vi "all_stages - state_machine.vi"() -> ()   [LabVIEW 2024]
uses:
  O:/DSG/Tyler/EIC/DIRC/daq/automated/Thorlabs.MotionControl.Controls.dll
  Thorlabs.MotionControl.Controls.dll
  O:/DSG/Tyler/EIC/DIRC/daq/automated/Thorlabs.MotionControl.IntegratedStepperMotorsCLI.dll
  Thorlabs.MotionControl.IntegratedStepperMotorsCLI.dll
  O:/DSG/Tyler/EIC/DIRC/daq/automated/Thorlabs.MotionControl.Benchtop.StepperMotorCLI.dll
  Thorlabs.MotionControl.Benchtop.StepperMotorCLI.dll
  <instrlib>/Keithley 6517/Keithley 6517.lvlib
panel:
  out "main-stage-refs":T1
  out "state-queue":T2(array[cluster])
  in  "build-seq":bool
  in  "PDA":dbl=85.0 format="%#_13g"
  in  "BMA":dbl=45.0 format="%#_13g"
  in  "BarY":dbl=150.0 format="%#_13g"
  in  "BarX":dbl=300.0 format="%#_13g"
  in  "PDY":dbl=150.0 format="%#_13g"
  in  "PDX":dbl=300.0 format="%#_13g"
  out "bypass-confirm":bool
  out "ySeq_hist":dbl[][](array[numeric])
  out "xSeq_hist":dbl[][](array[numeric])
  out "xSeq_diff":dbl[](array[numeric])
  out "ySeq_diff":dbl[](array[numeric])
  out "ySeq_in":dbl[](array[numeric])
  out "xSeq_in":dbl[](array[numeric])
  out "ySeq_res":dbl[](array[numeric])
  out "xSeq_res":dbl[](array[numeric])
  in  "go_seq_test":bool
  out "PD Values":cluster{"PD1":dbl, "PD2":dbl, "PD3":dbl}
  out "last-PD":dbl[](array[numeric])=[1.0, 1.0, 1.0]
  in  "move-bar":bool
  in  "mode-select":T3(radio) caption="Mode Select"
  in  "auto-align-grid":bool
  in  "auto-delta":dbl=0.5
  out "max value":dbl
  out "xOut":dbl
  out "yOut":dbl
  out "max indexes":i32[](array[numeric])
  in  "k":dbl=25.0
  in  "N trials":dbl=16.0
  in  "auto-align":bool
  out "pd_angle":dbl
  out "brewster_angle":dbl
  out "meter-visa":refnum<visa-resource-name>
  out "loop-rate":u32
  out "meter-stat":bool caption="Log Status"
  out "file-stat":bool caption="Log Status"
  out "stage-stat":bool caption="Log Status"
  out "last-save-time":string caption="Time of Last Save:"
  out "pd_y_pos":dbl
  out "pd_x_pos":dbl
  out "bar_y_pos":dbl
  out "bar_x_pos":dbl
  in  "nSamples":dbl=50.0 caption="# Samples"
  out "Current Time:":string
  in  "save-data":bool
  in  "bar-note":bool
  out "pd3_v":dbl caption="PD 3" format="%#.4g"
  out "pd2_v":dbl caption="PD 2" format="%#.4g"
  out "pd1_v":dbl caption="PD 1" format="%#.4g"
  out "meter-error":errorcluster
  out "log-error":errorcluster
  out "log-path":path caption="Path Data Will Save To:"
  out "start-msg":string
  out "stage-error":errorcluster
  in  "PD Angle":refnum<k24>(container)
  in  "Brewster":refnum<k24>(container)
  in  "PD Y":refnum<k24>(container)
  in  "PD X":refnum<k24>(container)
  in  "BAR Y":refnum<k24>(container)
  in  "stop":bool
  in  "BAR X":refnum<k24>(container)
  out "pd-plt":cluster{"[0]":dbl, "[1]":dbl, "[2]":dbl}(graph) caption="Measurement History"
  # "EXPERT DEBUGGING INFO"
  # "A"
  # "A"
  # "A"
  # "Work In Progress - please do not use"
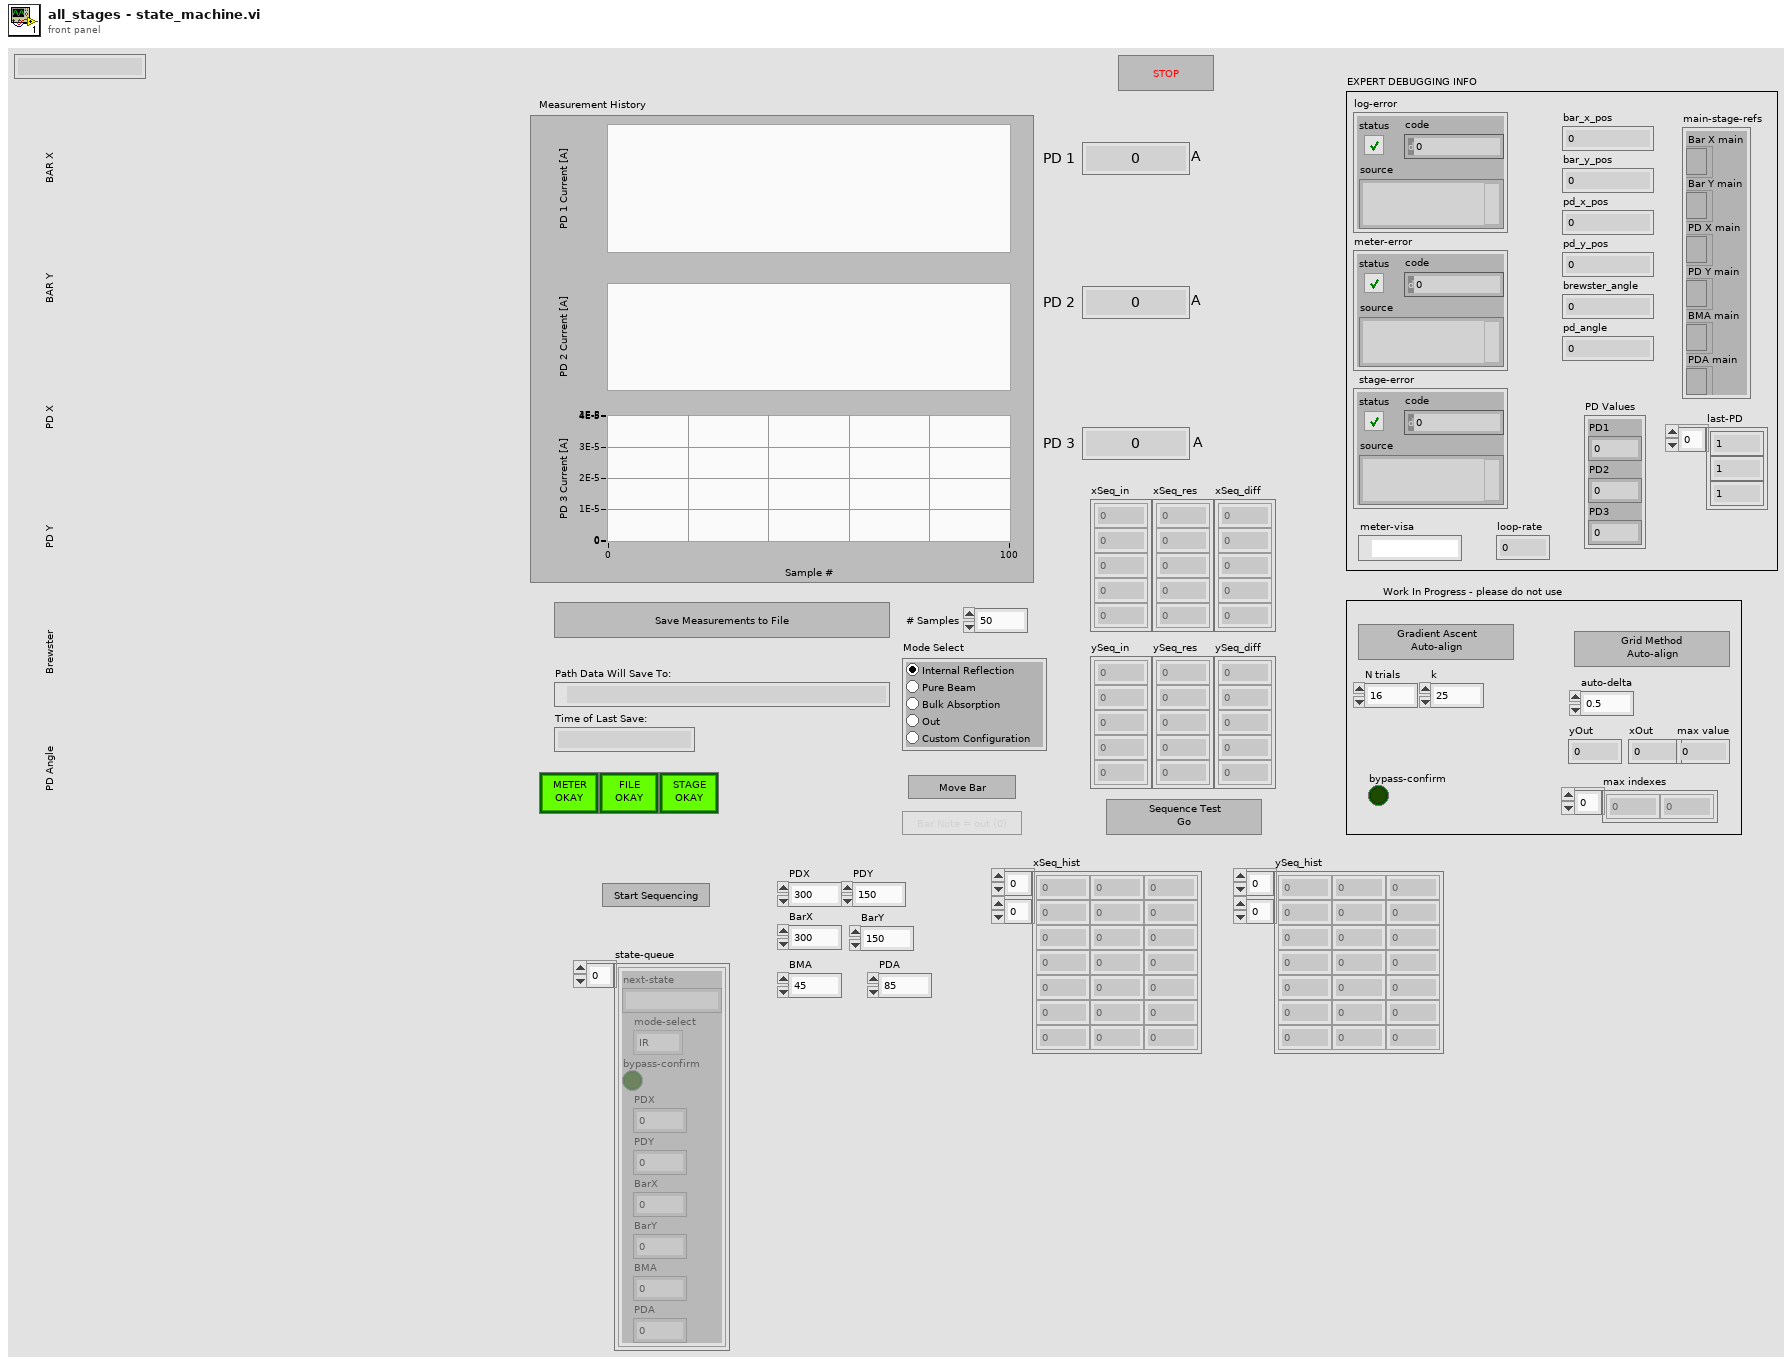
[diagram p1: front panel]
types:
  T1 = cluster{"Bar X main":refnum<k24>, "Bar Y main":refnum<k24>, "PD X main":refnum<k24>, "PD Y main":refnum<k24>, "BMA main":refnum<k24>, "PDA main":refnum<k24>}
  T2 = cluster{"next-state":string, "mode-select":enum32{"IR", "Pure", "Bulk", "Bar Out", "custom"}, "bypass-confirm":bool, "PDX":dbl, "PDY":dbl, "BarX":dbl, "BarY":dbl, "BMA":dbl, "PDA":dbl}[]
  T3 = enum32{"IR", "Pure", "Bulk", "Bar Out", "custom"}
  T4 = cluster{"Bar X":refnum<k24>, "Bar Y":refnum<k24>, "PD X":refnum<k24>, "PD Y":refnum<k24>, "Brewster":refnum<k24>, "PD Angle":refnum<k24>}
  T5 = enum16{"open", "replace", "create", "open or create", "replace or create", "replace or create with confirmation"}
  T6 = cluster{"next-state":string, "mode-select":enum32{"IR", "Pure", "Bulk", "Bar Out", "custom"}, "bypass-confirm":bool, "PDX":dbl, "PDY":dbl, "BarX":dbl, "BarY":dbl, "BMA":dbl, "PDA":dbl}
  T7 = cluster{"error":bool, "code":i32, "source":string}
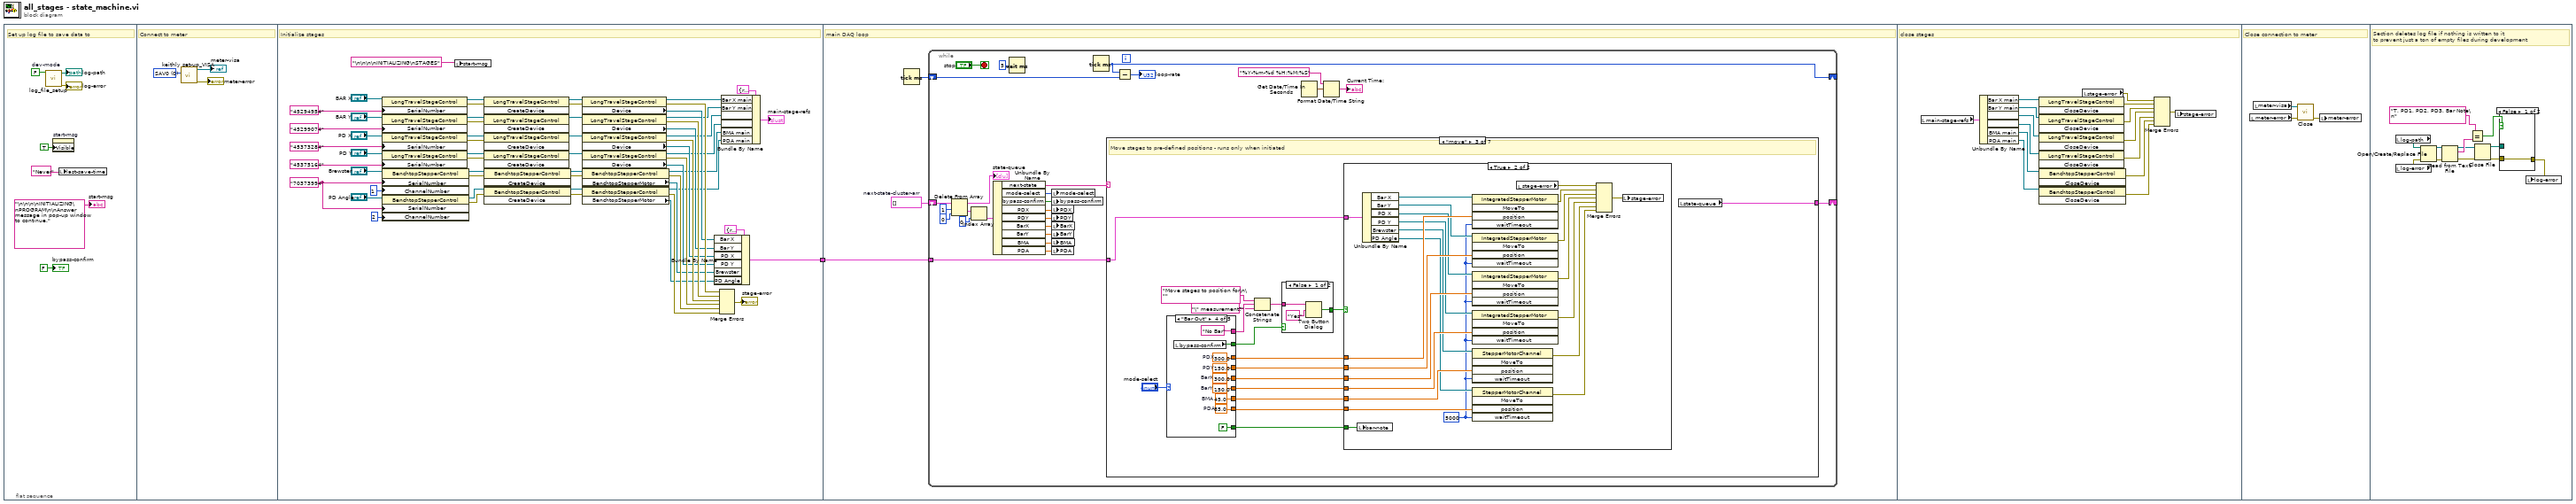
[diagram p0: block diagram]
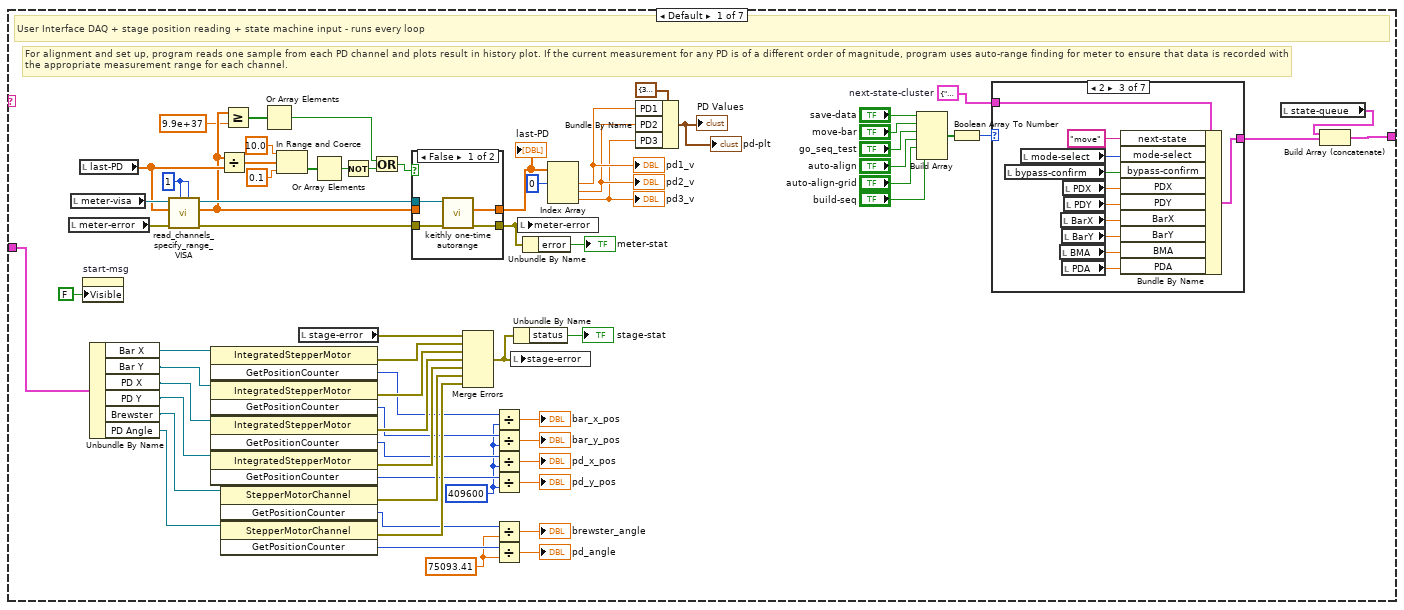
[diagram p2: hidden frame]
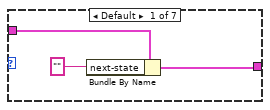
[diagram p3: hidden frame]
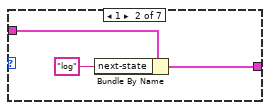
[diagram p4: hidden frame]
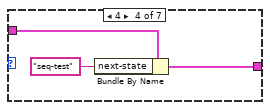
[diagram p5: hidden frame]
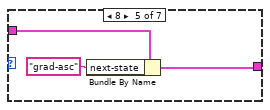
[diagram p6: hidden frame]
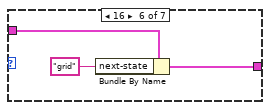
[diagram p7: hidden frame]
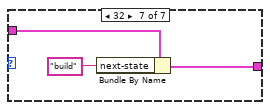
[diagram p8: hidden frame]
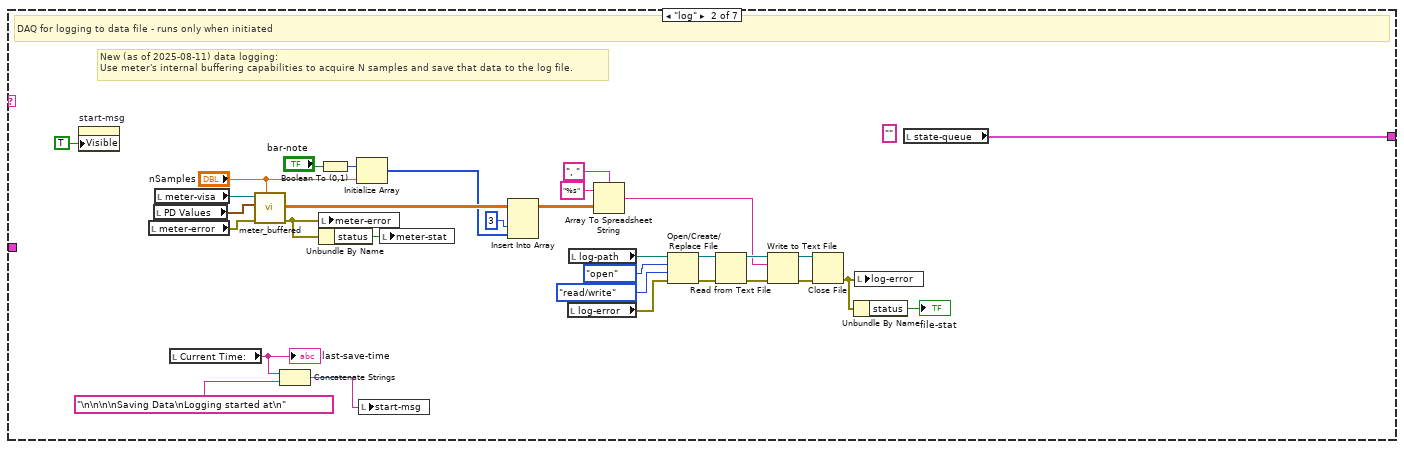
[diagram p10: hidden frame]
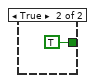
[diagram p11: hidden frame]
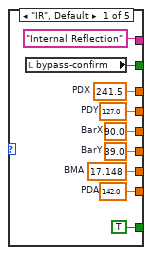
[diagram p12: hidden frame]
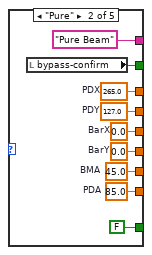
[diagram p13: hidden frame]
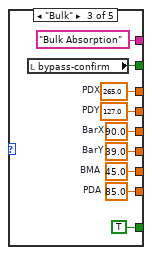
[diagram p14: hidden frame]
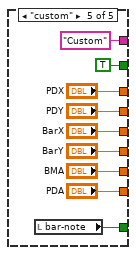
[diagram p15: hidden frame]
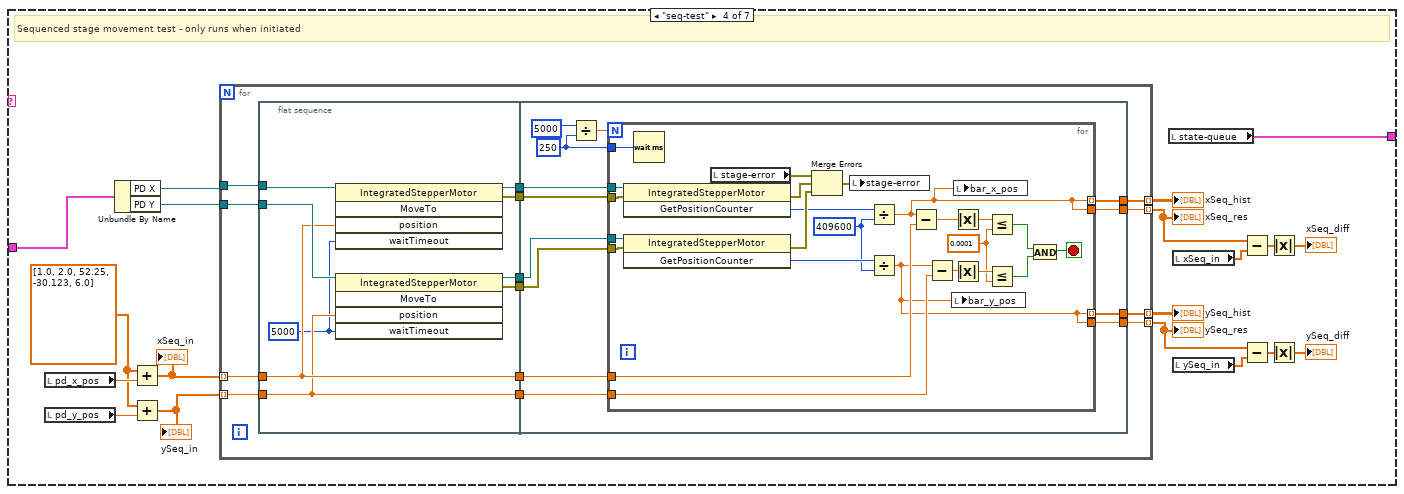
[diagram p17: hidden frame]
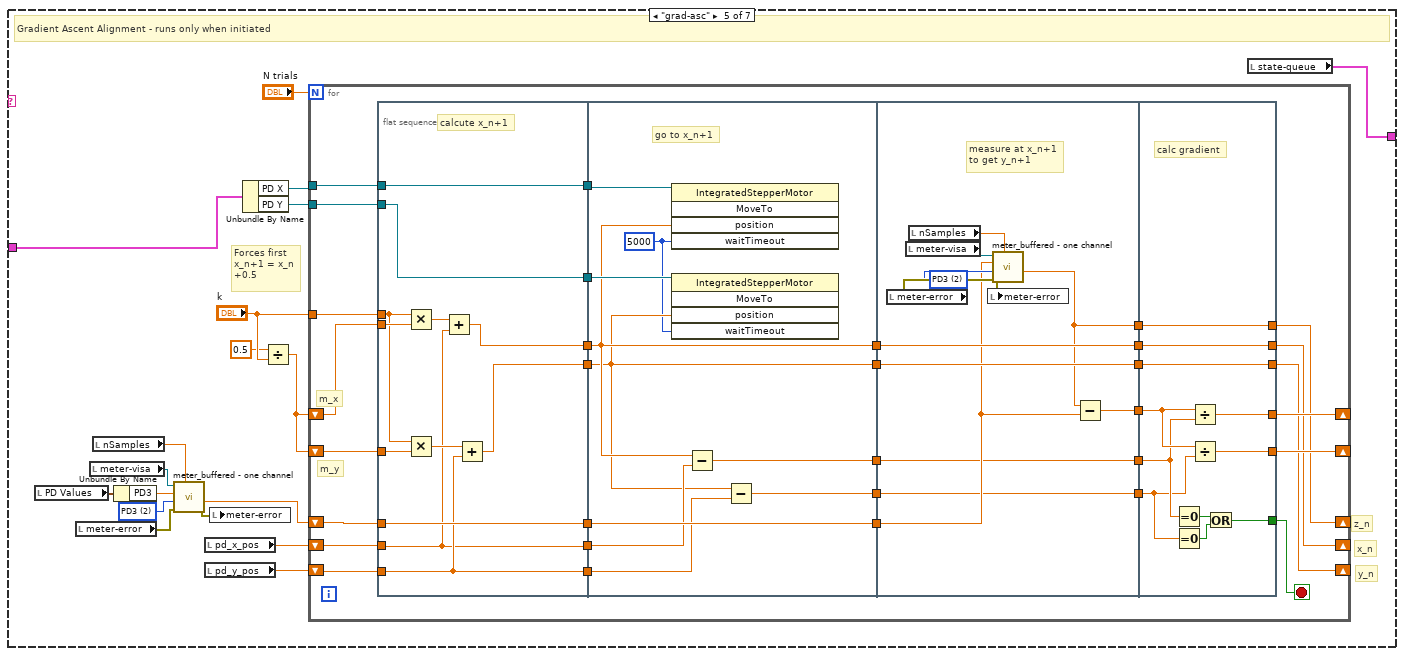
[diagram p18: hidden frame]
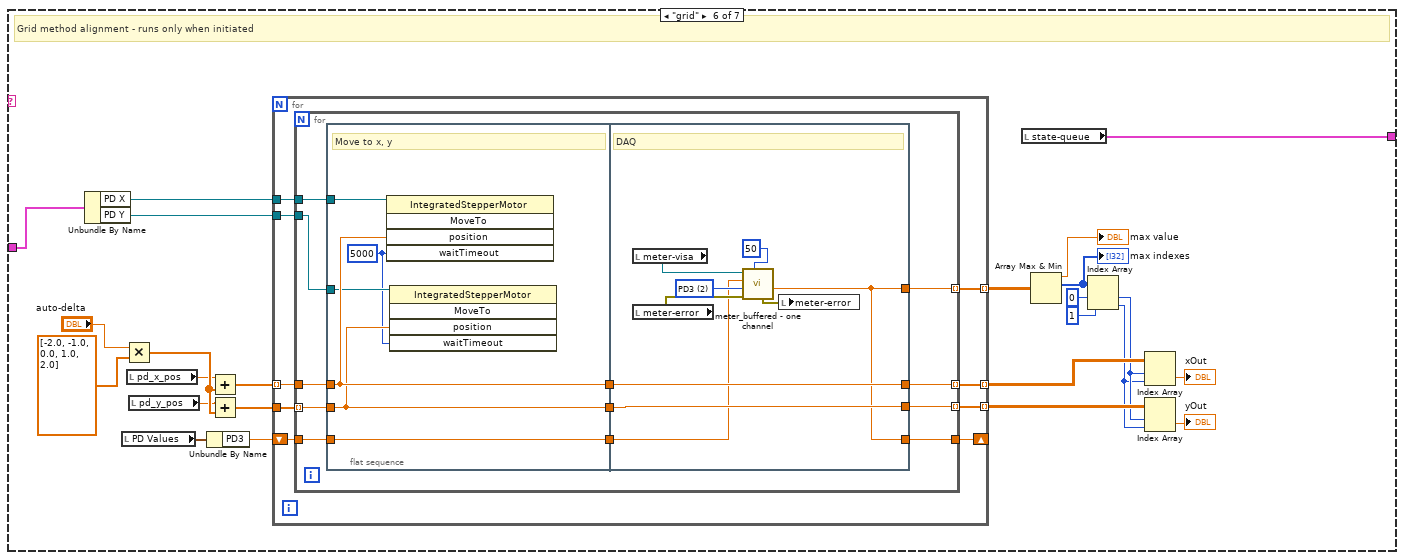
[diagram p19: hidden frame]
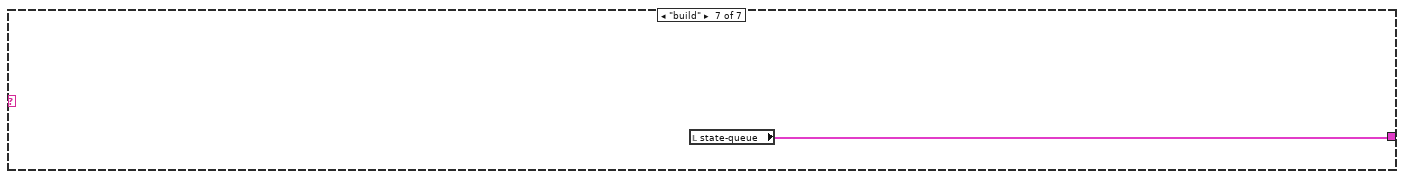
[diagram p20: hidden frame]
diagram:
  n1 = flat-sequence {
    tunnel: [w20] -> w1
    tunnel: w1 -> [w71]
    frame #0 {
      w8 = FALSE  # dev-mode
      # "Set up log file to save data to"
      n2 = call "log_file_setup.vi"("dev-mode"=w8) -> ("error out"=→"log-error":errorcluster, "appended path"=→"log-path":path)  [unwired: 8 in, 1 out]
      n3 = property on="start-msg" class="Str"("Visible"=TRUE) -> ()  [unwired: 2 in, 2 out]
      n4 = local write "last-save-time"("Never" ("date/time string")) -> ()
      "start-msg" <- "\n\n\n\nINITIALIZING\nPROGRAM\n\nAnswer message in pop-up window to continue." ("String")
      "bypass-confirm" <- FALSE
    }
    frame #1 {
      w9 = i16 0 items=["SAV0", "SAV1", "SAV2", "SAV3", "SAV4", "SAV5", "SAV6", "SAV7", "SAV8", "SAV9", "RST", "Preset"] ("ConfigOpt")
      # "Connect to meter"
      n5 = call "keithly set-up_VISA.vi"("ConfigOpt"=w9) -> ("error out"=→"meter-error":errorcluster, "meter-VISA"=→"meter-visa":refnum<visa-resource-name>)  [unwired: 9 in]
    }
    frame #2 {
      w28 = "70373994" ("SerialNumber")
      # "Initialize stages"
      n6 = property class="LongTravelStageControl"(reference="BAR X", "SerialNumber"="45294954") -> (reference out=w31:refnum<k24>, error out=w38:errorcluster)  [unwired: 1 in]
      n7 = property class="LongTravelStageControl"(reference="BAR Y", "SerialNumber"="45299074") -> (reference out=w32:refnum<k24>, error out=w39:errorcluster)  [unwired: 1 in]
      n8 = property class="LongTravelStageControl"(reference="PD X", "SerialNumber"="45373284") -> (reference out=w35:refnum<k24>, error out=w40:errorcluster)  [unwired: 1 in]
      n9 = property class="LongTravelStageControl"(reference="PD Y", "SerialNumber"="45375164") -> (reference out=w36:refnum<k24>, error out=w41:errorcluster)  [unwired: 1 in]
      n10 = property class="BenchtopStepperControl"(reference="Brewster", "SerialNumber"=w28, "ChannelNumber"=1) -> (reference out=w54:refnum<k24>, error out=w55:errorcluster)  [unwired: 1 in]
      n11 = property class="BenchtopStepperControl"(reference="PD Angle", "SerialNumber"=w28, "ChannelNumber"=2) -> (reference out=w53:refnum<k24>, error out=w56:errorcluster)  [unwired: 1 in]
      n12 = local write "start-msg"("\n\n\n\nINITIALIZING\nSTAGES" ("String")) -> ()
      n13 = invoke class="LongTravelStageControl" method="CreateDevice"(reference=w31, error in=w38) -> (reference out=w44:refnum<k24>, error out=w48:errorcluster)  [unwired: 1 in, 1 out]
      n14 = invoke class="LongTravelStageControl" method="CreateDevice"(reference=w32, error in=w39) -> (reference out=w45:refnum<k24>)  [unwired: 1 in, 2 out]
      n15 = invoke class="LongTravelStageControl" method="CreateDevice"(reference=w35, error in=w40) -> (reference out=w46:refnum<k24>)  [unwired: 1 in, 2 out]
      n16 = invoke class="LongTravelStageControl" method="CreateDevice"(reference=w36, error in=w41) -> (reference out=w47:refnum<k24>)  [unwired: 1 in, 2 out]
      n17 = invoke class="BenchtopStepperControl" method="CreateDevice"(reference=w54, error in=w55) -> (reference out=w51:refnum<k24>, error out=w49:errorcluster)  [unwired: 1 in, 1 out]
      n18 = invoke class="BenchtopStepperControl" method="CreateDevice"(reference=w53, error in=w56) -> (reference out=w50:refnum<k24>, error out=w52:errorcluster)  [unwired: 1 in, 1 out]
      n19 = property class="LongTravelStageControl"(reference=w44, error in=w48) -> (reference out=w18:refnum<k24>, error out=w68:errorcluster, "Device"=w57:refnum<k24>)
      n20 = property class="LongTravelStageControl"(reference=w45) -> (reference out=w17:refnum<k24>, error out=w63:errorcluster, "Device"=w58:refnum<k24>)  [unwired: 1 in]
      n21 = property class="LongTravelStageControl"(reference=w46) -> (reference out=w16:refnum<k24>, error out=w64:errorcluster, "Device"=w59:refnum<k24>)  [unwired: 1 in]
      n22 = property class="LongTravelStageControl"(reference=w47) -> (reference out=w15:refnum<k24>, error out=w65:errorcluster, "Device"=w60:refnum<k24>)  [unwired: 1 in]
      n23 = property class="BenchtopStepperControl"(reference=w51, error in=w49) -> (reference out=w14:refnum<k24>, error out=w66:errorcluster, "BenchtopStepperMotor"=w61:refnum<k24>)
      n24 = property class="BenchtopStepperControl"(reference=w50, error in=w52) -> (reference out=w13:refnum<k24>, error out=w67:errorcluster, "BenchtopStepperMotor"=w62:refnum<k24>)
      n25 = Bundle By Name(cluster=T4 {"Bar X"=refnum, "Bar Y"=refnum, "PD X"=refnum, "PD Y"=refnum, "Brewster"=refnum, "PD Angle"=refnum}, "Bar X"=w57, "Bar Y"=w58, "PD X"=w59, "PD Y"=w60, "Brewster"=w61, "PD Angle"=w62) -> (w20:T4)
      n26 = Merge Errors(w68, w63, w64, w65, w66, w67) -> (→"stage-error":errorcluster)
      n27 = Bundle By Name(cluster=T1 {"Bar X main"=refnum, "Bar Y main"=refnum, "PD X main"=refnum, "PD Y main"=refnum, "BMA main"=refnum, "PDA main"=refnum}, "Bar X main"=w18, "Bar Y main"=w17, "PD X main"=w16, "PD Y main"=w15, "BMA main"=w14, "PDA main"=w13) -> (→"main-stage-refs":T1)
    }
    frame #3 {
      w70 = T2 []  # next-state-cluster-arr
      # "main DAQ loop"
      n28 = Tick Count (ms)() -> (millisecond timer value=w72:u32)
      n29 = while {
        shift-right: [w97] -> _
        shift-left: w72 -> [w96]
        tunnel: w71 -> [w94]
        shift-right: [w73] -> _
        shift-left: w70 -> [w76]
        stop <- "stop" stop-if-true
        n30 = Delete From Array(array=w76, length=1, index=0) -> (deleted portion=w74:T2, array with subset deleted=→"state-queue":T2)
        n31 = Index Array(array=w74, index=0) -> (element=w86:T6)
        n32 = Unbundle By Name(w86) -> ("next-state"=w85:string, "mode-select"=w77:T3, "bypass-confirm"=w78:bool, "PDX"=w84:dbl, "PDY"=w83:dbl, "BarX"=w82:dbl, "BarY"=w81:dbl, "BMA"=w80:dbl, "PDA"=w79:dbl)
        n33 = Wait (ms)(milliseconds to wait=u32 5) -> ()  [unwired: 1 out]
        n34 = local write "mode-select"(w77) -> ()
        n35 = local write "bypass-confirm"(w78) -> ()
        n36 = local write "PDX"(w84) -> ()
        n37 = local write "PDY"(w83) -> ()
        n38 = local write "BarX"(w82) -> ()
        n39 = local write "BarY"(w81) -> ()
        n40 = local write "BMA"(w80) -> ()
        n41 = local write "PDA"(w79) -> ()
        n42 = Tick Count (ms)() -> (millisecond timer value=w97:u32)
        n43 = case shown="\"move\"" w85 {
          tunnel: w94 -> [w159 _ w237 w339 w417 w520 _]
          tunnel: [w101 w203 w235 w323 w402 w497 w557] -> w73
          frame Default {
            w100 = T6 {"next-state"="", "mode-select"=enum."IR", "bypass-confirm"=FALSE, "PDX"=300.0, "PDY"=150.0, "BarX"=300.0, "BarY"=150.0, "BMA"=45.0, "PDA"=85.0}  # next-state-cluster
            w129 = u32 1 ("preDAQ  wait ms")
            w138 = 75093.41 ("GetPositionCounter")
            w139 = 409600 ("y")
            # "For alignment and set up, program reads one sample from each PD channel and plots result in history plot. If the current measurement for any PD is of a different order of magnitude, program uses auto-range finding for meter to ensure that data is recorded with the appropriate measurement range for each channel."
            # "User Interface DAQ + stage position reading + state machine input - runs every loop"
            n44 = local read "meter-error"() -> (w130:errorcluster)
            n45 = local read "meter-visa"() -> (w131:refnum<visa-resource-name>)
            n46 = local read "last-PD"() -> (w121:dbl[])
            n47 = property on="start-msg" class="Str"("Visible"=FALSE) -> ()  [unwired: 2 in, 2 out]
            n48 = Unbundle By Name(w159) -> ("Bar X"=w158:refnum<k24>, "Bar Y"=w157:refnum<k24>, "PD X"=w156:refnum<k24>, "PD Y"=w155:refnum<k24>, "Brewster"=w154:refnum<k24>, "PD Angle"=w153:refnum<k24>)
            n49 = call "read_channels_specify_range_VISA.vi"("postDAQ  wait ms"=w129, "preDAQ  wait ms"=w129, "error in"=w130, "range"=w121, "VISA resource in"=w131) -> ("error out"=w123:T7, "data"=w107:dbl[], "VISA resource out"=w122:refnum<visa-resource-name>)  [unwired: 4 in]
            n50 = invoke class="IntegratedStepperMotor" method="GetPositionCounter"(reference=w158) -> (error out=w151:errorcluster, "GetPositionCounter"=w145:i32)  [unwired: 2 in, 1 out]
            n51 = invoke class="IntegratedStepperMotor" method="GetPositionCounter"(reference=w157) -> (error out=w150:errorcluster, "GetPositionCounter"=w144:i32)  [unwired: 2 in, 1 out]
            n52 = invoke class="IntegratedStepperMotor" method="GetPositionCounter"(reference=w156) -> (error out=w149:errorcluster, "GetPositionCounter"=w143:i32)  [unwired: 2 in, 1 out]
            n53 = invoke class="IntegratedStepperMotor" method="GetPositionCounter"(reference=w155) -> (error out=w148:errorcluster, "GetPositionCounter"=w142:i32)  [unwired: 2 in, 1 out]
            n54 = Divide(x=w107, y=w121) -> (x/y=w126:dbl[])
            n55 = invoke class="StepperMotorChannel" method="GetPositionCounter"(reference=w154) -> (error out=w147:errorcluster, "GetPositionCounter"=w141:i32)  [unwired: 2 in, 1 out]
            n56 = invoke class="StepperMotorChannel" method="GetPositionCounter"(reference=w153) -> (error out=w146:errorcluster, "GetPositionCounter"=w140:i32)  [unwired: 2 in, 1 out]
            n57 = Greater Or Equal?(x=w107, y=9.9e+37) -> (x >= y?=w105:bool[])
            n58 = Or Array Elements(Boolean array=w105) -> (logical OR=w104:bool)
            n59 = In Range and Coerce(upper limit=10.0, x=w126, lower limit=0.1) -> (In Range?=w124:bool[])  [unwired: 1 out]
            n60 = local read "stage-error"() -> (w152:errorcluster)
            n61 = Or Array Elements(Boolean array=w124) -> (logical OR=w125:bool)
            n62 = Not(x=w125) -> (.not. x?=w109:bool)
            n63 = Or(x=w104, y=w109) -> (x .or. y?=w108:bool)
            n64 = case shown="False" w108 {
              tunnel: w123 -> [w200 w202]
              tunnel: [w199 w202] -> w165
              tunnel: [w198 w201] -> w160
              tunnel: w107 -> [_ w201]
              tunnel: w122 -> [w197 _]
              frame False {
                n65 = call "keithly one-time autorange.vi"("error in"=w200, "VISA in"=w197) -> ("error out"=w199:errorcluster, "data"=w198:dbl[])  [unwired: 7 in, 1 out]
              }
              frame True {
              }
            }
            "last-PD" <- w160
            n66 = Merge Errors(w152, w151, w150, w149, w148, w147, w146) -> (w118:errorcluster)
            n67 = Divide(x=w145, y=w139) -> (x/y=→"bar_x_pos":dbl)
            n68 = Divide(x=w144, y=w139) -> (x/y=→"bar_y_pos":dbl)
            n69 = Divide(x=w143, y=w139) -> (x/y=→"pd_x_pos":dbl)
            n70 = Divide(x=w142, y=w139) -> (x/y=→"pd_y_pos":dbl)
            n71 = Divide(x=w141, y=w138) -> (x/y=→"brewster_angle":dbl)
            n72 = Divide(x=w140, y=w138) -> (x/y=→"pd_angle":dbl)
            n73 = local write "stage-error"(w118) -> ()
            n74 = Unbundle By Name(w118) -> ("status"=→"stage-stat":bool)
            n75 = local write "meter-error"(w165) -> ()
            n76 = Unbundle By Name(w165) -> ("error"=→"meter-stat":bool)
            n77 = Index Array(array=w160, index #1=0 ("index")) -> (element #1=w163:dbl, element #2=w162:dbl, element #3=w161:dbl)  [unwired: 2 in]
            "pd3_v" <- w161
            "pd2_v" <- w162
            "pd1_v" <- w163
            n78 = Bundle By Name(cluster=cluster{"PD1":dbl, "PD2":dbl, "PD3":dbl} {"PD1"=3e-05, "PD2"=3e-05, "PD3"=3e-05} ("PD ranges"), "PD1"=w163, "PD2"=w162, "PD3"=w161) -> (→"pd-plt" →"PD Values":cluster{"PD1":dbl, "PD2":dbl, "PD3":dbl})
            n79 = Build Array("save-data", "move-bar", "go_seq_test", "auto-align", "auto-align-grid", "build-seq") -> (w112:bool[])
            n80 = Boolean Array To Number(Boolean array=w112) -> (number=w111:u32)
            n81 = case shown="2" w111 {
              tunnel: w100 -> [w170 w173 w184 w187 w190 w193 w196]
              tunnel: [w168 w171 w182 w185 w188 w191 w194] -> w99
              frame Default {
                n82 = Bundle By Name(cluster=w170, "next-state"="") -> (w168:T6)
              }
              frame 1 {
                n83 = Bundle By Name(cluster=w173, "next-state"="log") -> (w171:T6)
              }
              frame 2 {
                n84 = local read "bypass-confirm"() -> (w175:bool)
                n85 = local read "mode-select"() -> (w174:T3)
                n86 = local read "BMA"() -> (w180:dbl)
                n87 = local read "BarX"() -> (w178:dbl)
                n88 = local read "BarY"() -> (w179:dbl)
                n89 = local read "PDA"() -> (w181:dbl)
                n90 = local read "PDX"() -> (w176:dbl)
                n91 = local read "PDY"() -> (w177:dbl)
                n92 = Bundle By Name(cluster=w184, "next-state"="move", "mode-select"=w174, "bypass-confirm"=w175, "PDX"=w176, "PDY"=w177, "BarX"=w178, "BarY"=w179, "BMA"=w180, "PDA"=w181) -> (w182:T6)
              }
              frame 4 {
                n93 = Bundle By Name(cluster=w187, "next-state"="seq-test") -> (w185:T6)
              }
              frame 8 {
                n94 = Bundle By Name(cluster=w190, "next-state"="grad-asc") -> (w188:T6)
              }
              frame 16 {
                n95 = Bundle By Name(cluster=w193, "next-state"="grid") -> (w191:T6)
              }
              frame 32 {
                n96 = Bundle By Name(cluster=w196, "next-state"="build") -> (w194:T6)
              }
            }
            n97 = local read "state-queue"() -> (w102:T2)
            n98 = Build Array (concatenate)(w102, w99) -> (w101:T2)
          }
          frame "log" {
            (unwired) ""
            # "New (as of 2025-08-11) data logging:\nUse meter's internal buffering capabilities to acquire N samples and save that data to the log file."
            # "DAQ for logging to data file - runs only when initiated"
            n99 = property on="start-msg" class="Str"("Visible"=TRUE) -> ()  [unwired: 2 in, 2 out]
            n100 = local read "meter-error"() -> (w233:errorcluster)
            n101 = local read "PD Values"() -> (w208:cluster{"PD1":dbl, "PD2":dbl, "PD3":dbl})
            n102 = local read "meter-visa"() -> (w234:refnum<visa-resource-name>)
            n103 = local read "Current Time:"() -> (w206:string)
            "last-save-time" <- w206
            n104 = call "meter_buffered.vi"("Samples"="nSamples", "error in"=w233, "PD ranges"=w208, "meter-VISA"=w234) -> ("error out"=w209:errorcluster, "ch1-3 data"=w221:dbl[][])  [unwired: 5 in, 1 out]
            n105 = Concatenate Strings(w206, "\n\n\n\nSaving Data\nLogging started at\n" ("String")) -> (w204:string)
            n106 = local write "meter-error"(w209) -> ()
            n107 = Unbundle By Name(w209) -> ("status"=w210:bool)
            n108 = Boolean To (0,1)(Boolean="bar-note") -> (0, 1=w218:i16)
            n109 = Initialize Array(w218, "nSamples") -> (w219:i16[])
            n110 = local write "start-msg"(w204) -> ()
            n111 = local write "meter-stat"(w210) -> ()
            n112 = Insert Into Array(array=w221, index (col)=3 ("disabled index (col)"), new element=w219) -> (w215:dbl[][])  [unwired: 1 in]
            n113 = local read "log-error"() -> (w231:errorcluster)
            n114 = local read "log-path"() -> (w232:path)
            n115 = Array To Spreadsheet String(delimiter (Tab)=", ", array=w215, 3:"%s" ("format string")) -> (spreadsheet string=w214:string)
            n116 = Open/Create/Replace File(file path (use dialog)=w232, error in=w231, operation (0:open)=T5."open", access (0:read/write)=enum16{"read/write", "read-only", "write-only"}."read/write") -> (refnum out=w230:refnum<file>, error out=w226:errorcluster)  [unwired: 2 in, 1 out]
            n117 = Read from Text File(file (use dialog)=w230, error in=w226) -> (refnum out=w227:refnum<file>, error out=w225:errorcluster)  [unwired: 2 in, 2 out]
            n118 = Write to Text File(file (use dialog)=w227, text=w214, error in=w225) -> (refnum out=w229:refnum<file>, error out=w228:errorcluster)  [unwired: 1 in, 1 out]
            n119 = Close File(refnum=w229, error in=w228) -> (error out=w224:errorcluster)  [unwired: 1 out]
            n120 = Unbundle By Name(w224) -> ("status"=→"file-stat":bool)
            n121 = local write "log-error"(w224) -> ()
            n122 = local read "state-queue"() -> (w203:T2)
          }
          frame "move" {
            # "Move stages to pre-defined positions - runs only when initiated"
            n123 = case shown="\"Bar Out\"" "mode-select" {
              tunnel: [w263 w272 w281 w290 "PDX"] -> w249
              tunnel: [w258 w271 w280 w289 "PDY"] -> w248
              tunnel: [w259 w270 w279 w288 "BarX"] -> w247
              tunnel: [w260 w269 w278 w287 "BarY"] -> w246
              tunnel: [w261 w268 w277 w286 "BMA"] -> w245
              tunnel: [w262 w267 w276 w285 "PDA"] -> w244
              tunnel: [TRUE FALSE TRUE FALSE w292] -> w243
              tunnel: ["Internal Reflection" "Pure Beam" "Bulk Absorption" "No Bar" "Custom"] -> w241
              tunnel: [w255 w264 w273 w282 TRUE ("bypass-confirm")] -> w236
              frame "IR", Default {
                w262 = 142.0  # PDA
                w258 = 127.0  # PDY
                w263 = 241.5  # PDX
                w260 = 39.0  # BarY
                w259 = 90.0  # BarX
                w261 = 17.148  # BMA
                n124 = local read "bypass-confirm"() -> (w255:bool)
              }
              frame "Pure" {
                w267 = 85.0  # PDA
                w271 = 127.0  # PDY
                w272 = 265.0  # PDX
                w269 = 0.0  # BarY
                w270 = 0.0  # BarX
                w268 = 45.0  # BMA
                n125 = local read "bypass-confirm"() -> (w264:bool)
              }
              frame "Bulk" {
                w276 = 85.0  # PDA
                w280 = 127.0  # PDY
                w281 = 265.0  # PDX
                w278 = 39.0  # BarY
                w279 = 90.0  # BarX
                w277 = 45.0  # BMA
                n126 = local read "bypass-confirm"() -> (w273:bool)
              }
              frame "Bar Out" {
                w285 = 85.0  # PDA
                w289 = 150.0  # PDY
                w290 = 300.0  # PDX
                w287 = 150.0  # BarY
                w288 = 300.0  # BarX
                w286 = 45.0  # BMA
                n127 = local read "bypass-confirm"() -> (w282:bool)
              }
              frame "custom" {
                n128 = local read "bar-note"() -> (w292:bool)
              }
            }
            n129 = Concatenate Strings("Move stages to position for\n\"", w241, "\" measurement?" ("string")) -> (w239:string)
            n130 = case shown="False" w236 {
              tunnel: [w253 TRUE ("T button?")] -> w242
              tunnel: w239 -> [w252 _]
              frame False {
                n131 = Two Button Dialog(message=w252, 2:"Yes" ("T button name (\"OK\")")) -> (T button?=w253:bool)  [unwired: 1 in]
              }
              frame True {
              }
            }
            n132 = case shown="True" w242 {
              tunnel: w249 -> [_ w314]
              tunnel: w248 -> [_ w313]
              tunnel: w247 -> [_ w312]
              tunnel: w246 -> [_ w311]
              tunnel: w245 -> [_ w310]
              tunnel: w244 -> [_ w309]
              tunnel: w243 -> [_ w308]
              tunnel: w237 -> [_ w307]
              frame False {
              }
              frame True {
                w300 = 5000 ("waitTimeout")
                n133 = local write "bar-note"(w308) -> ()
                n134 = Unbundle By Name(w307) -> ("Bar X"=w306:refnum<k24>, "Bar Y"=w301:refnum<k24>, "PD X"=w302:refnum<k24>, "PD Y"=w303:refnum<k24>, "Brewster"=w304:refnum<k24>, "PD Angle"=w305:refnum<k24>)
                n135 = invoke class="IntegratedStepperMotor" method="MoveTo"(reference=w306, "position"=w314, "waitTimeout"=w300) -> (error out=w321:errorcluster)  [unwired: 2 in, 4 out]
                n136 = invoke class="IntegratedStepperMotor" method="MoveTo"(reference=w301, "position"=w313, "waitTimeout"=w300) -> (error out=w320:errorcluster)  [unwired: 2 in, 4 out]
                n137 = invoke class="IntegratedStepperMotor" method="MoveTo"(reference=w302, "position"=w312, "waitTimeout"=w300) -> (error out=w319:errorcluster)  [unwired: 2 in, 4 out]
                n138 = invoke class="IntegratedStepperMotor" method="MoveTo"(reference=w303, "position"=w311, "waitTimeout"=w300) -> (error out=w318:errorcluster)  [unwired: 2 in, 4 out]
                n139 = invoke class="StepperMotorChannel" method="MoveTo"(reference=w304, "position"=w310, "waitTimeout"=w300) -> (error out=w317:errorcluster)  [unwired: 2 in, 4 out]
                n140 = invoke class="StepperMotorChannel" method="MoveTo"(reference=w305, "position"=w309, "waitTimeout"=w300) -> (error out=w316:errorcluster)  [unwired: 2 in, 4 out]
                n141 = local read "stage-error"() -> (w322:errorcluster)
                n142 = Merge Errors(w322, w321, w320, w319, w318, w317, w316) -> (w315:errorcluster)
                n143 = local write "stage-error"(w315) -> ()
              }
            }
            n144 = local read "state-queue"() -> (w235:T2)
          }
          frame "seq-test" {
            w335 = dbl[] [1.0, 2.0, 52.25, -30.123, 6.0]
            # "Sequenced stage movement test - only runs when initiated"
            n145 = local read "pd_x_pos"() -> (w341:dbl)
            n146 = local read "pd_y_pos"() -> (w340:dbl)
            n147 = Unbundle By Name(w339) -> ("PD X"=w338:refnum<k24>, "PD Y"=w337:refnum<k24>)
            n148 = Add(x=w335, y=w341) -> (x+y=w336:dbl[])
            "xSeq_in" <- w336
            n149 = Add(x=w335, y=w340) -> (x+y=w334:dbl[])
            "ySeq_in" <- w334
            n150 = for {
              tunnel: w338 -> [w351]
              tunnel: w337 -> [w350]
              tunnel: w336 -> [w343] mode=indexing
              tunnel: w334 -> [w349] mode=indexing
              tunnel: [w348] -> w324 mode=indexing
              tunnel: [w347] -> w331 mode=indexing
              tunnel: [w346] -> w327 mode=indexing
              tunnel: [w345] -> w326 mode=indexing
              n151 = flat-sequence {
                tunnel: [w364] -> w355
                tunnel: [w363] -> w354
                tunnel: [w362] -> w353
                tunnel: [w361] -> w352
                tunnel: w350 -> [w359]
                tunnel: w351 -> [w360]
                tunnel: w349 -> [w357]
                tunnel: [w358] -> w344
                tunnel: w343 -> [w358]
                tunnel: [w357] -> w342
                tunnel: w352 -> [w373]
                tunnel: w353 -> [w375]
                tunnel: w354 -> [w374]
                tunnel: w355 -> [w376]
                tunnel: [w366] -> w348
                tunnel: [w365] -> w347
                tunnel: [w367] -> w346
                tunnel: [w368] -> w345
                tunnel: w344 -> [w370]
                tunnel: w342 -> [w369]
                frame #0 {
                  w356 = 5000 ("waitTimeout")
                  n152 = invoke class="IntegratedStepperMotor" method="MoveTo"(reference=w360, "position"=w358, "waitTimeout"=w356) -> (reference out=w364:refnum<k24>, error out=w362:errorcluster)  [unwired: 2 in, 3 out]
                  n153 = invoke class="IntegratedStepperMotor" method="MoveTo"(reference=w359, "position"=w357, "waitTimeout"=w356) -> (reference out=w363:refnum<k24>, error out=w361:errorcluster)  [unwired: 2 in, 3 out]
                }
                frame #1 {
                  w372 = 250
                  n154 = Divide(x=5000, y=w372) -> (x/y=w371:dbl)
                  n155 = for {
                    N: w371 -> [_]
                    tunnel: w370 -> [w386]
                    tunnel: w369 -> [w385]
                    tunnel: w376 -> [w384]
                    tunnel: w375 -> [w383]
                    tunnel: w374 -> [w382]
                    tunnel: w373 -> [w381]
                    tunnel: w372 -> [w380]
                    tunnel: [w378] -> w368 mode=indexing
                    tunnel: [w379] -> w367 mode=indexing
                    tunnel: [w379] -> w366
                    tunnel: [w378] -> w365
                    stop <- w387 stop-if-true
                    w390 = 0.0001 ("y")
                    w395 = 409600 ("y")
                    n156 = invoke class="IntegratedStepperMotor" method="GetPositionCounter"(reference=w384, error in=w383) -> (error out=w399:errorcluster, "GetPositionCounter"=w397:i32)  [unwired: 1 in, 1 out]
                    n157 = invoke class="IntegratedStepperMotor" method="GetPositionCounter"(reference=w382, error in=w381) -> (error out=w398:errorcluster, "GetPositionCounter"=w396:i32)  [unwired: 1 in, 1 out]
                    n158 = Wait (ms)(milliseconds to wait=w380) -> ()  [unwired: 1 out]
                    n159 = local read "stage-error"() -> (w401:errorcluster)
                    n160 = Merge Errors(w401, w399, w398) -> (w400:errorcluster)
                    n161 = local write "stage-error"(w400) -> ()
                    n162 = Divide(x=w397, y=w395) -> (x/y=w379:dbl)
                    n163 = Divide(x=w396, y=w395) -> (x/y=w378:dbl)
                    n164 = Subtract(x=w379, y=w386) -> (x-y=w394:dbl)
                    n165 = Subtract(x=w378, y=w385) -> (x-y=w393:dbl)
                    n166 = local write "bar_y_pos"(w378) -> ()
                    n167 = Absolute Value(x=w394) -> (abs(x)=w392:dbl)
                    n168 = Absolute Value(x=w393) -> (abs(x)=w391:dbl)
                    n169 = local write "bar_x_pos"(w379) -> ()
                    n170 = Less Or Equal?(x=w392, y=w390) -> (x <= y?=w389:bool)
                    n171 = Less Or Equal?(x=w391, y=w390) -> (x <= y?=w388:bool)
                    n172 = And(x=w389, y=w388) -> (x .and. y?=w387:bool)
                  }
                }
              }
            }
            "xSeq_res" <- w324
            "ySeq_res" <- w331
            "xSeq_hist" <- w327
            "ySeq_hist" <- w326
            n173 = local read "state-queue"() -> (w323:T2)
            n174 = local read "xSeq_in"() -> (w325:dbl[])
            n175 = local read "ySeq_in"() -> (w328:dbl[])
            n176 = Subtract(x=w324, y=w325) -> (x-y=w333:dbl[])
            n177 = Subtract(x=w331, y=w328) -> (x-y=w330:dbl[])
            n178 = Absolute Value(x=w333) -> (abs(x)=→"xSeq_diff":dbl[])
            n179 = Absolute Value(x=w330) -> (abs(x)=→"ySeq_diff":dbl[])
          }
          frame "grad-asc" {
            w412 = u16 2 items=["PD1", "PD2", "PD3"] ("Photodiode Select")
            # "y_n"
            # "x_n"
            # "z_n"
            # "Forces first x_n+1 = x_n +0.5"
            # "Gradient Ascent Alignment - runs only when initiated"
            n180 = local read "PD Values"() -> (w406:cluster{"PD1":dbl, "PD2":dbl, "PD3":dbl})
            n181 = local read "meter-error"() -> (w410:errorcluster)
            n182 = local read "meter-visa"() -> (w409:refnum<visa-resource-name>)
            n183 = local read "nSamples"() -> (w407:dbl)
            n184 = Unbundle By Name(w406) -> ("PD3"=w405:dbl)
            n185 = call "meter_buffered - one channel.vi"("Samples"=w407, "error in"=w410, "Channel"=w412, "PD Range"=w405, "meter-VISA"=w409) -> ("error out"=w411:errorcluster, "avg"=w408:dbl)  [unwired: 3 in, 2 out]
            n186 = local read "pd_x_pos"() -> (w419:dbl)
            n187 = local read "pd_y_pos"() -> (w418:dbl)
            n188 = local write "meter-error"(w411) -> ()
            n189 = Unbundle By Name(w417) -> ("PD X"=w404:refnum<k24>, "PD Y"=w403:refnum<k24>)
            n190 = Divide(x=0.5, y="k") -> (x/y=w416:dbl)
            n191 = for {
              N: "N trials" -> [_]
              shift-right: [w434] -> _
              shift-left: w419 -> [w446]
              shift-right: [w435] -> _
              shift-left: w408 -> [w447]
              tunnel: "k" -> [w451]
              shift-right: [w433] -> _
              shift-left: w418 -> [w443]
              shift-right: [w438] -> _
              shift-left: w416 -> [w436]
              shift-right: [w439] -> _
              shift-left: w416 -> [w437]
              tunnel: w404 -> [w428]
              tunnel: w403 -> [w426]
              stop <- w429 stop-if-true
              # "m_y"
              # "m_x"
              n192 = flat-sequence {
                tunnel: w451 -> [w458]
                tunnel: [w463] -> w450
                tunnel: w447 -> [w462]
                tunnel: [w462] -> w448
                tunnel: w446 -> [w452]
                tunnel: [w452] -> w445
                tunnel: [w454] -> w444
                tunnel: w443 -> [w454]
                tunnel: [w461] -> w442
                tunnel: w437 -> [w460]
                tunnel: w436 -> [w459]
                tunnel: w428 -> [w457]
                tunnel: [w457] -> w427
                tunnel: w426 -> [w456]
                tunnel: [w456] -> w425
                tunnel: [w466] -> w432
                tunnel: [w473] -> w431
                tunnel: [w465] -> w430
                tunnel: [w472] -> w423
                tunnel: [w471] -> w420
                tunnel: w425 -> [w469]
                tunnel: w427 -> [w470]
                tunnel: w442 -> [w465]
                tunnel: w444 -> [w467]
                tunnel: w445 -> [w468]
                tunnel: w448 -> [w473]
                tunnel: w450 -> [w466]
                tunnel: w432 -> [w485]
                tunnel: [w485] -> w449
                tunnel: w431 -> [w478]
                tunnel: w430 -> [w484]
                tunnel: [w484] -> w441
                tunnel: [w479] -> w440
                tunnel: [w477] -> w424
                tunnel: w423 -> [w476]
                tunnel: [w476] -> w422
                tunnel: [w475] -> w421
                tunnel: w420 -> [w475]
                tunnel: w449 -> [w494]
                tunnel: [w494] -> w434
                tunnel: w441 -> [w493]
                tunnel: [w493] -> w433
                tunnel: w440 -> [w492]
                tunnel: [w492] -> w435
                tunnel: [w496] -> w439
                tunnel: [w495] -> w438
                tunnel: [w489] -> w429
                tunnel: w424 -> [w488]
                tunnel: w422 -> [w487]
                tunnel: w421 -> [w486]
                frame #0 {
                  # "calcute x_n+1"
                  n193 = Multiply(x=w458, y=w460) -> (x*y=w453:dbl)
                  n194 = Multiply(x=w458, y=w459) -> (x*y=w455:dbl)
                  n195 = Add(x=w453, y=w452) -> (x+y=w463:dbl)
                  n196 = Add(x=w455, y=w454) -> (x+y=w461:dbl)
                }
                frame #1 {
                  w464 = 5000 ("waitTimeout")
                  # "go to x_n+1"
                  n197 = invoke class="IntegratedStepperMotor" method="MoveTo"(reference=w470, "position"=w466, "waitTimeout"=w464) -> ()  [unwired: 2 in, 5 out]
                  n198 = invoke class="IntegratedStepperMotor" method="MoveTo"(reference=w469, "position"=w465, "waitTimeout"=w464) -> ()  [unwired: 2 in, 5 out]
                  n199 = Subtract(x=w466, y=w468) -> (x-y=w472:dbl)
                  n200 = Subtract(x=w465, y=w467) -> (x-y=w471:dbl)
                }
                frame #2 {
                  w480 = u16 2 items=["PD1", "PD2", "PD3"] ("Photodiode Select")
                  # "measure at x_n+1\nto get y_n+1"
                  n201 = local read "meter-error"() -> (w482:errorcluster)
                  n202 = local read "meter-visa"() -> (w483:refnum<visa-resource-name>)
                  n203 = local read "nSamples"() -> (w474:dbl)
                  n204 = call "meter_buffered - one channel.vi"("Samples"=w474, "error in"=w482, "Channel"=w480, "PD Range"=w478, "meter-VISA"=w483) -> ("error out"=w481:errorcluster, "avg"=w479:dbl)  [unwired: 3 in, 2 out]
                  n205 = local write "meter-error"(w481) -> ()
                  n206 = Subtract(x=w479, y=w478) -> (x-y=w477:dbl)
                }
                frame #3 {
                  # "calc gradient"
                  n207 = Equal To 0?(x=w487) -> (x = 0?=w491:bool)
                  n208 = Equal To 0?(x=w486) -> (x = 0?=w490:bool)
                  n209 = Divide(x=w488, y=w487) -> (x/y=w496:dbl)
                  n210 = Divide(x=w488, y=w486) -> (x/y=w495:dbl)
                  n211 = Or(x=w491, y=w490) -> (x .or. y?=w489:bool)
                }
              }
            }
            n212 = local read "state-queue"() -> (w402:T2)
          }
          frame "grid" {
            # "Grid method alignment - runs only when initiated"
            n213 = Unbundle By Name(w520) -> ("PD X"=w499:refnum<k24>, "PD Y"=w498:refnum<k24>)
            n214 = local read "PD Values"() -> (w505:cluster{"PD1":dbl, "PD2":dbl, "PD3":dbl})
            n215 = Multiply(x="auto-delta", y=dbl[] [-2.0, -1.0, 0.0, 1.0, 2.0]) -> (x*y=w506:dbl[])
            n216 = local read "pd_x_pos"() -> (w503:dbl)
            n217 = local read "pd_y_pos"() -> (w502:dbl)
            n218 = Unbundle By Name(w505) -> ("PD3"=w504:dbl)
            n219 = Add(x=w503, y=w506) -> (x+y=w509:dbl[])
            n220 = Add(x=w502, y=w506) -> (x+y=w508:dbl[])
            n221 = for {
              tunnel: w509 -> [w528] mode=indexing
              tunnel: w508 -> [w529]
              tunnel: [w527] -> w516 mode=indexing
              tunnel: [w526] -> w517 mode=indexing
              tunnel: [w525] -> w511 mode=indexing
              tunnel: w499 -> [w524]
              tunnel: w498 -> [w523]
              shift-right: [w521] -> _
              shift-left: w504 -> [w522]
              n222 = for {
                tunnel: w529 -> [w541] mode=indexing
                tunnel: w528 -> [w540]
                tunnel: [w539] -> w526 mode=indexing
                tunnel: [w538] -> w527 mode=indexing
                tunnel: [w537] -> w525 mode=indexing
                tunnel: w524 -> [w534]
                tunnel: w523 -> [w533]
                tunnel: w522 -> [w532]
                tunnel: [w530] -> w521
                n223 = flat-sequence {
                  tunnel: w541 -> [w543]
                  tunnel: w540 -> [w546]
                  tunnel: [w546] -> w536
                  tunnel: [w543] -> w535
                  tunnel: w534 -> [w547]
                  tunnel: w533 -> [w545]
                  tunnel: w532 -> [w544]
                  tunnel: [w544] -> w531
                  tunnel: [w556] -> w539
                  tunnel: [w555] -> w538
                  tunnel: [w548] -> w537
                  tunnel: [w548] -> w530
                  tunnel: w531 -> [w549]
                  tunnel: w535 -> [w555]
                  tunnel: w536 -> [w556]
                  frame #0 {
                    w542 = 5000 ("waitTimeout")
                    # "Move to x, y"
                    n224 = invoke class="IntegratedStepperMotor" method="MoveTo"(reference=w547, "position"=w546, "waitTimeout"=w542) -> ()  [unwired: 2 in, 5 out]
                    n225 = invoke class="IntegratedStepperMotor" method="MoveTo"(reference=w545, "position"=w543, "waitTimeout"=w542) -> ()  [unwired: 2 in, 5 out]
                  }
                  frame #1 {
                    w551 = u16 2 items=["PD1", "PD2", "PD3"] ("Photodiode Select")
                    # "DAQ"
                    n226 = local read "meter-visa"() -> (w554:refnum<visa-resource-name>)
                    n227 = local read "meter-error"() -> (w553:errorcluster)
                    n228 = call "meter_buffered - one channel.vi"("Samples"=u32 50 ("preDAQ  wait ms"), "error in"=w553, "Channel"=w551, "PD Range"=w549, "meter-VISA"=w554) -> ("error out"=w552:errorcluster, "avg"=w548:dbl)  [unwired: 3 in, 2 out]
                    n229 = local write "meter-error"(w552) -> ()
                  }
                }
              }
            }
            n230 = local read "state-queue"() -> (w497:T2)
            n231 = Array Max & Min(array=w511) -> (max value=→"max value":dbl, max index (indices)=w513:i32[])  [unwired: 2 out]
            "max indexes" <- w513
            n232 = Index Array(array=w513, index #1=0 ("index"), index #2=1 ("index")) -> (element #1=w501:i32, element #2=w500:i32)
            n233 = Index Array(array=w517, index (row)=w501, index (col)=w500) -> (element=→"xOut":dbl)
            n234 = Index Array(array=w516, index (row)=w501, index (col)=w500) -> (element=→"yOut":dbl)
          }
          frame "build" {
            n235 = local read "state-queue"() -> (w557:T2)
          }
        }
        n236 = Subtract(x=w97, y=w96) -> (x-y=→"loop-rate":u32)
        n237 = Get Date/Time In Seconds() -> (seconds since 1Jan1904=w92:timestamp)
        n238 = Format Date/Time String(time format string (%c)="%Y-%m-%d %H:%M:%S", seconds (now)=w92) -> (date/time string=→"Current Time:":string)  [unwired: 1 in]
      }
    }
    frame #4 {
      # "close stages"
      n239 = local read "main-stage-refs"() -> (w558:T1)
      n240 = Unbundle By Name(w558) -> ("Bar X main"=w564:refnum<k24>, "Bar Y main"=w563:refnum<k24>, "PD X main"=w562:refnum<k24>, "PD Y main"=w561:refnum<k24>, "BMA main"=w560:refnum<k24>, "PDA main"=w559:refnum<k24>)
      n241 = invoke class="LongTravelStageControl" method="CloseDevice"(reference=w564) -> (error out=w565:errorcluster)  [unwired: 2 in, 2 out]
      n242 = invoke class="LongTravelStageControl" method="CloseDevice"(reference=w563) -> (error out=w566:errorcluster)  [unwired: 2 in, 2 out]
      n243 = invoke class="LongTravelStageControl" method="CloseDevice"(reference=w562) -> (error out=w567:errorcluster)  [unwired: 2 in, 2 out]
      n244 = invoke class="LongTravelStageControl" method="CloseDevice"(reference=w561) -> (error out=w568:errorcluster)  [unwired: 2 in, 2 out]
      n245 = invoke class="BenchtopStepperControl" method="CloseDevice"(reference=w560) -> (error out=w569:errorcluster)  [unwired: 2 in, 2 out]
      n246 = invoke class="BenchtopStepperControl" method="CloseDevice"(reference=w559) -> (error out=w570:errorcluster)  [unwired: 2 in, 2 out]
      n247 = local read "stage-error"() -> (w571:errorcluster)
      n248 = Merge Errors(w571, w565, w566, w567, w568, w569, w570) -> (w572:errorcluster)
      n249 = local write "stage-error"(w572) -> ()
    }
    frame #5 {
      # "Close connection to meter"
      n250 = local read "meter-error"() -> (w574:errorcluster)
      n251 = local read "meter-visa"() -> (w573:refnum<visa-resource-name>)
      n252 = call <instrlib>:"Close.vi"("error in (no error)"=w574, "VISA resource name"=w573) -> ("error out"=w575:errorcluster)  [unwired: 9 in]
      n253 = local write "meter-error"(w575) -> ()
    }
    frame #6 {
      # "Section deletes log file if nothing is written to it\nto prevent just a ton of empty files during development"
      n254 = local read "log-path"() -> (w577:path)
      n255 = local read "log-error"() -> (w582:errorcluster)
      n256 = Open/Create/Replace File(file path (use dialog)=w577, error in=w582) -> (refnum out=w587:refnum<file>, error out=w586:errorcluster)  [unwired: 4 in, 1 out]
      n257 = Read from Text File(file (use dialog)=w587, error in=w586) -> (refnum out=w584:refnum<file>, text=w585:string, error out=w583:errorcluster)  [unwired: 2 in, 1 out]
      n258 = Equal?(x="T, PD1, PD2, PD3, Bar Note\n" ("Display"), y=w585) -> (x = y?=w581:bool)
      n259 = Close File(refnum=w584, error in=w583) -> (path=w580:path, error out=w579:errorcluster)
      n260 = case shown="False" w581 {
        tunnel: w580 -> [_ w591]
        tunnel: w579 -> [w588 w590]
        tunnel: [w588 w589] -> w578
        frame False {
        }
        frame True {
          n261 = Delete(path (use dialog)=w591, error in=w590) -> (error out=w589:errorcluster)  [unwired: 3 in, 2 out]
        }
      }
      n262 = local write "log-error"(w578) -> ()
    }
  }
